vi "Check Custom Shortcuts.vi"(7 "All Possible Shortcuts":string[](array[string]), 11 "Item Text":string) -> (2 "Shortcut":string, 3 "Name":string)   [LabVIEW 2021, in "Seq Edit Quick Drop.lvlib"]
uses:
  Seq Edit Quick Drop.lvlib
  <vilib>/regexp/Match Regular Expression.xnode
  <vilib>/Utility/error.llb/whitespace.ctl
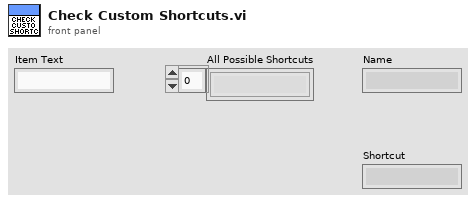
[diagram p1: front panel]
types:
  T1 = typedef "whitespace.ctl" = u16
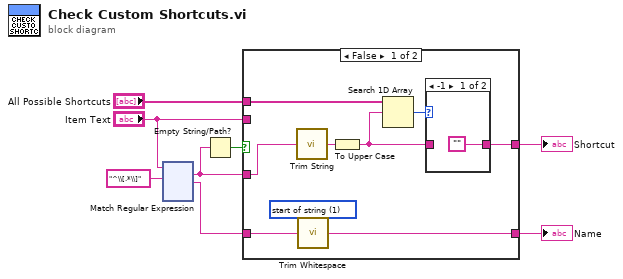
[diagram p0: block diagram]
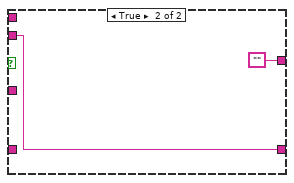
[diagram p3: hidden frame]
diagram:
  n1 = xnode "Match Regular Expression"("input string"="Item Text", "regular expression"="^\\[.*\\]") -> ("whole match"=w2:string, "after match"=w3:string)  [unwired: 4 in, 3 out]
  n2 = Empty String/Path?(string/path=w2) -> (empty?=w7:bool)
  n3 = case shown="False" w7 {
    tunnel: "Item Text" -> [_ w21]
    tunnel: [w15 w21] -> w5
    tunnel: [w12 ""] -> w4
    tunnel: w3 -> [w17 _]
    tunnel: w2 -> [w14 _]
    tunnel: "All Possible Shortcuts" -> [w9 _]
    frame False {
      w16 = T1 1 items=["both", "start of string", "end of string"] ("location (both)")
      n4 = call "Trim String.vi"("String In"=w14) -> ("String Out"=w11:string)
      n5 = call <vilib>:"Trim Whitespace.vi"("string"=w17, "location (both)"=w16) -> ("trimmed string"=w15:string)
      n6 = To Upper Case(1:w11) -> (0:w10:string)
      n7 = Search 1D Array(1D array=w9, element=w10) -> (index of element=w13:i32)  [unwired: 1 in]
      n8 = case shown="-1" w13 {
        tunnel: ["" w19] -> w12
        tunnel: w10 -> [_ w19]
        frame -1 {
        }
        frame Default {
        }
      }
    }
    frame True {
    }
  }
  "Name" <- w5
  "Shortcut" <- w4
